vi "Test Update - Simple Case With Things In the Middle.vi"(11 "Test Case In":refnum<class "Camera Tests.lvclass">) -> (0 "error out":errorcluster, 3 "Test Case Out":refnum<class "Camera Tests.lvclass">)   [LabVIEW 2021, in "Camera Tests.lvclass"]
uses:
  Camera Tests.lvclass
  4993e8ee-a06a-463a-9684-69129f64d5ce.vi
  Application Specific/Camera/Camera.lvclass
  Re-use Libraries/Vector 2D/Vector 2D.lvclass
  e086f2d9-95d8-4aa4-9347-c0290e2d8edc.vi
  eae4dcd3-09e3-422e-aed5-3483da5873f4.vi
  46c90443-85e4-43eb-a6eb-fc75b5417668.vi
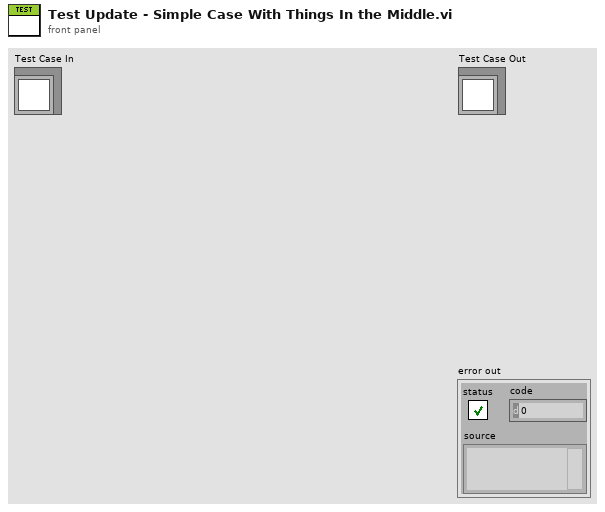
[diagram p1: front panel]
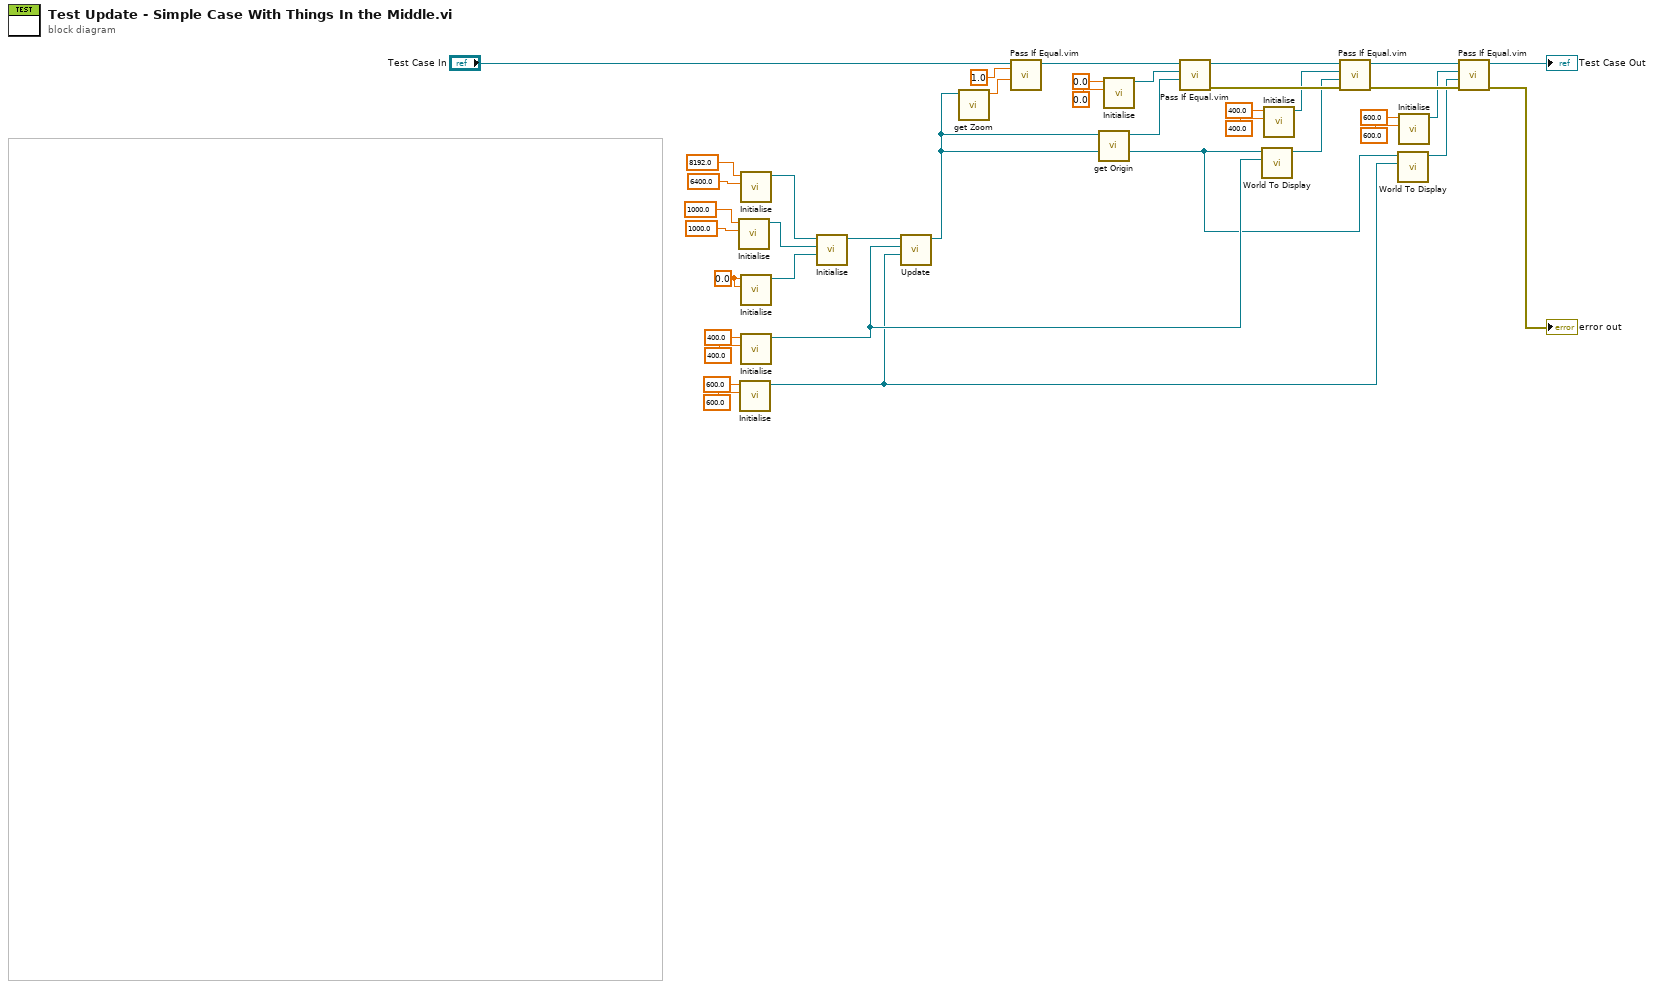
[diagram p0: block diagram]
diagram:
  w37 = sgl 0.0 ("x")
  n1 = call "Initialise.vi"("y"=sgl 1000.0 ("x"), "x"=sgl 1000.0) -> ("Vector 2D out"=w1:refnum<class "Vector 2D.lvclass">)  [unwired: 9 in]
  n2 = call "Initialise.vi"("y"=sgl 600.0, "x"=sgl 600.0) -> ("Vector 2D out"=w6:refnum<class "Vector 2D.lvclass">)  [unwired: 9 in]
  n3 = call "Initialise.vi"("y"=sgl 6400.0 ("x"), "x"=sgl 8192.0) -> ("Vector 2D out"=w38:refnum<class "Vector 2D.lvclass">)  [unwired: 9 in]
  n4 = call "Initialise.vi"("y"=w37, "x"=w37) -> ("Vector 2D out"=w36:refnum<class "Vector 2D.lvclass">)  [unwired: 9 in]
  n5 = call "Initialise.vi"("y"=sgl 400.0, "x"=sgl 400.0) -> ("Vector 2D out"=w24:refnum<class "Vector 2D.lvclass">)  [unwired: 9 in]
  n6 = call "Initialise.vi"("Origin"=w36, "View Size"=w1, "World Size"=w38) -> ("Camera out"=w31:refnum<class "Camera.lvclass">)  [unwired: 8 in]
  n7 = call "Update.vi"("Player 2 Position"=w6, "Player 1 Position"=w24, "Camera in"=w31) -> ("Camera out"=w7:refnum<class "Camera.lvclass">)  [unwired: 8 in]
  n8 = call "get Zoom.vi"("Camera in"=w7) -> ("Zoom Level"=w16:sgl)  [unwired: 10 in]
  n9 = call "Pass If Equal.vim"("Actual"=w16, "Expected"=sgl 1.0 ("Zoom Level"), "LUnit Test Case In"="Test Case In") -> ("LUnit Test Case Out"=w17:refnum<class "Camera Tests.lvclass">)  [unwired: 7 in, 1 out]
  n10 = call "get Origin.vi"("Camera in"=w7) -> ("Origin"=w30:refnum<class "Vector 2D.lvclass">)  [unwired: 10 in]
  n11 = call "Initialise.vi"("y"=sgl 0.0, "x"=sgl 0.0) -> ("Vector 2D out"=w27:refnum<class "Vector 2D.lvclass">)  [unwired: 9 in]
  n12 = call "Pass If Equal.vim"("Actual"=w30, "Expected"=w27, "LUnit Test Case In"=w17) -> ("error out"=w25:errorcluster, "LUnit Test Case Out"=w26:refnum<class "Camera Tests.lvclass">)  [unwired: 7 in]
  n13 = call "World To Display.vi"("World Position"=w24, "Camera in"=w7) -> ("Display Position"=w20:refnum<class "Vector 2D.lvclass">)  [unwired: 9 in]
  n14 = call "Initialise.vi"("y"=sgl 400.0, "x"=sgl 400.0) -> ("Vector 2D out"=w21:refnum<class "Vector 2D.lvclass">)  [unwired: 9 in]
  n15 = call "Pass If Equal.vim"("error in (no error)"=w25, "Actual"=w20, "Expected"=w21, "LUnit Test Case In"=w26) -> ("error out"=w12:errorcluster, "LUnit Test Case Out"=w14:refnum<class "Camera Tests.lvclass">)  [unwired: 6 in]
  n16 = call "World To Display.vi"("World Position"=w6, "Camera in"=w7) -> ("Display Position"=w5:refnum<class "Vector 2D.lvclass">)  [unwired: 9 in]
  n17 = call "Initialise.vi"("y"=sgl 600.0, "x"=sgl 600.0) -> ("Vector 2D out"=w8:refnum<class "Vector 2D.lvclass">)  [unwired: 9 in]
  n18 = call "Pass If Equal.vim"("error in (no error)"=w12, "Actual"=w5, "Expected"=w8, "LUnit Test Case In"=w14) -> ("error out"=→"error out":errorcluster, "LUnit Test Case Out"=→"Test Case Out":refnum<class "Camera Tests.lvclass">)  [unwired: 6 in]
